vi "Versioned Write.vi"(9 "Path Stuff":T10 {"?"."Limits"."StoopidFast (fps)" min=0.0; "?"."Limits"."Jerk (fps^3)" min=0.0 step=1.0; "?"."Limits"."Accel (fps^2)" min=0.0; "?"."Limits"."Velocity (fps)" min=0.0; "?"."Overrides"."Angle Override" step=5.0; "?"."Overrides"."Velocity Override" step=5.0; "?"."Overrides"."Angular Override" step=5.0; "?"."Angular Limits"."Jerk (deg/s^3)" min=0.0 step=1.0; "?"."Angular Limits"."Accel (deg/s^2)" min=0.0; "?"."Angular Limits"."Velocity (deg/s)" min=0.0}, 10 "Filename":string, 11 "Bordeaux paths in":path) -> ()   [LabVIEW 2025]
uses:
  Types/Trajectory Data.ctl
  Types/Segment Type.ctl
  Types/Single Cmd Info.ctl
  <vilib>/picture/picture.llb/imagedata.ctl
  Types/Limits.ctl
  Types/Overrides.ctl
  Types/Angluar Limits.ctl
  Types/Drive Type.ctl
  Types/Path Type.ctl
panel:
  in  "?":T11
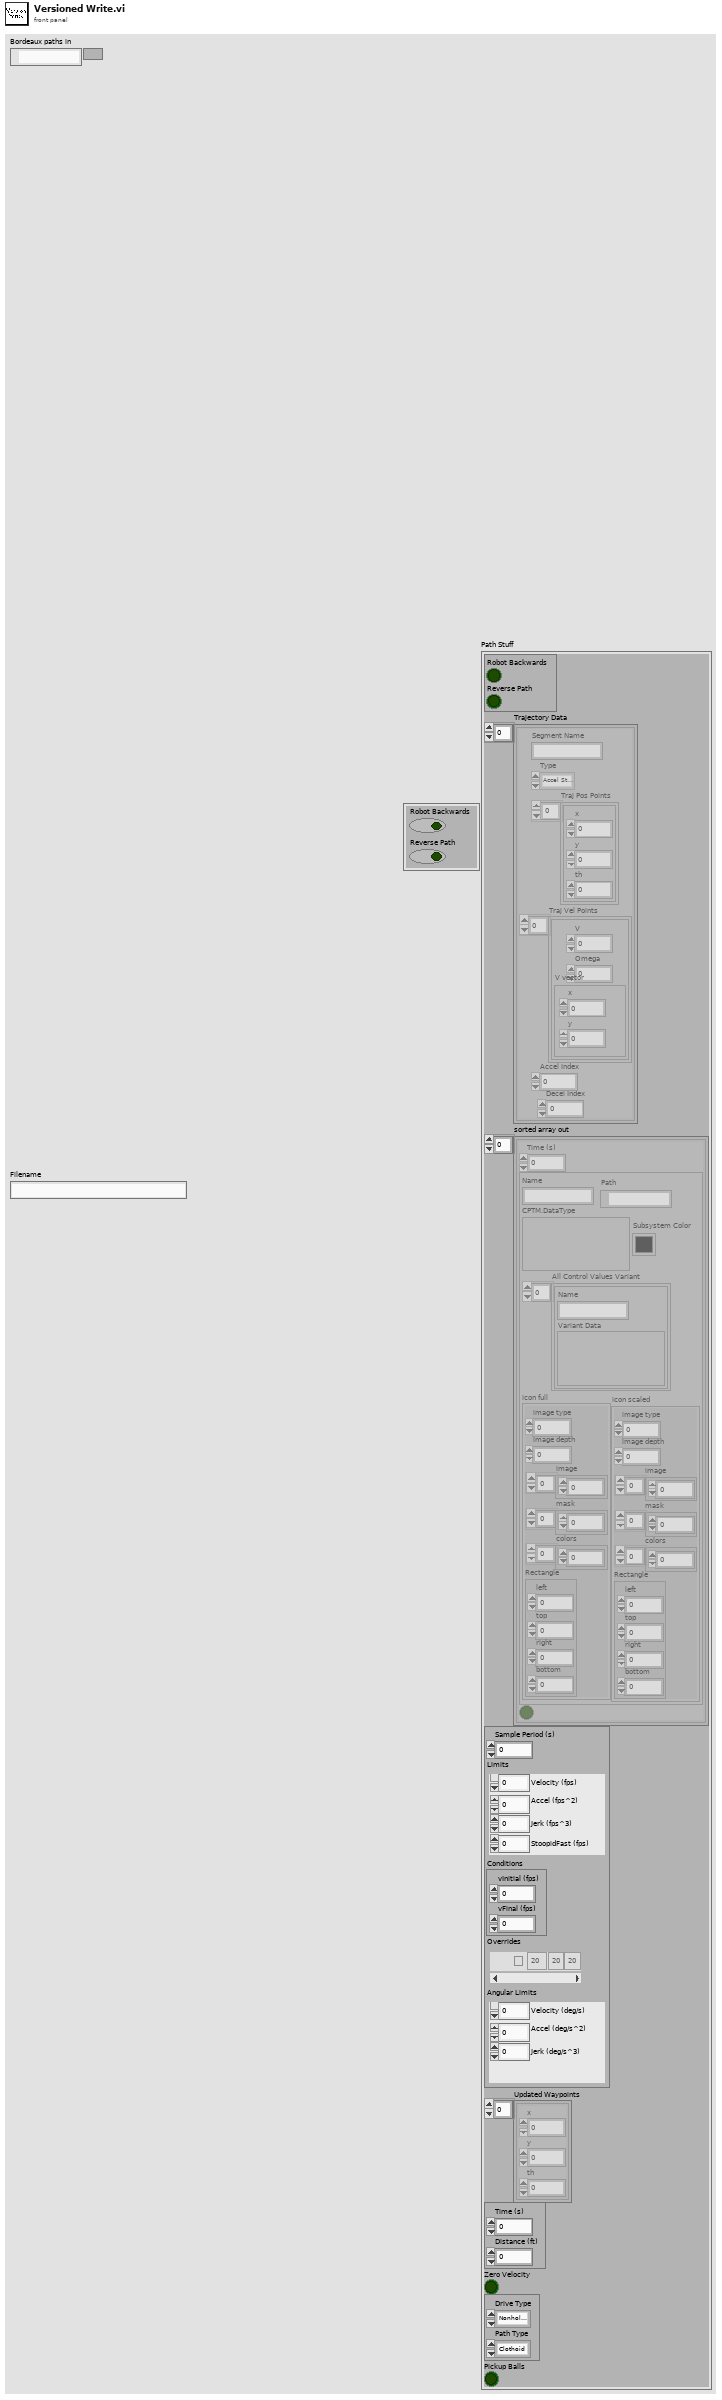
[diagram p1: front panel]
types:
  T1 = typedef "Trajectory Data.ctl" = cluster{"Segment Name":string, "Type":T2, "Traj Pos Points":cluster{"x":dbl, "y":dbl, "th":dbl}[], "Traj Vel Points":cluster{"V":dbl, "Omega":dbl, "V vector":cluster{"y":dbl, "x":dbl}}[], "Accel Index":i32, "Decel Index":i32}[]
  T2 = typedef "Segment Type.ctl" = enum16{"Accel Straight", "Const Straight", "Blend", "Circle", "Bezier"}
  T3 = typedef "Single Cmd Info.ctl" = cluster{"Name":string, "CPTM.DataType":variant, "All Control Values Variant":cluster{"Name":string, "Variant Data":variant}[], "icon full":T4, "icon scaled":T4, "Path":path, "Subsystem Color":u32}
  T4 = typedef "imagedata.ctl" = cluster{"image type":i32, "image depth":i32, "image":u8[], "mask":u8[], "colors":u32[], "Rectangle":cluster{"left":i16, "top":i16, "right":i16, "bottom":i16}}
  T5 = typedef "Limits.ctl" = cluster{"Velocity (fps)":dbl, "Accel (fps^2)":dbl, "Jerk (fps^3)":dbl, "StoopidFast (fps)":dbl}
  T6 = typedef "Overrides.ctl" = cluster{"Count":string, "Angular Override":dbl, "Enabled?":bool, "Velocity Override":dbl, "Angle Override":dbl}[]
  T7 = typedef "Angluar Limits.ctl" = cluster{"Velocity (deg/s)":dbl, "Accel (deg/s^2)":dbl, "Jerk (deg/s^3)":dbl}
  T8 = typedef "Drive Type.ctl" = enum16{"Nonholonomic", "Holonomic"}
  T9 = typedef "Path Type.ctl" = enum16{"Clothoid", "Bezier"}
  T10 = cluster{cluster{"Robot Backwards":bool, "Reverse Path":bool}, "Trajectory Data":T1, "sorted array out":cluster{"Time (s)":dbl, T3, bool}[], cluster{"Sample Period (s)":dbl, "Limits":T5, "Conditions":cluster{"vInitial (fps)":dbl, "vFinal (fps)":dbl}, "Overrides":T6, "Angular Limits":T7}, "Updated Waypoints":cluster{"x":dbl, "y":dbl, "th":dbl}[], cluster{"Time (s)":dbl, "Distance (ft)":dbl}, "Zero Velocity":bool, cluster{"Drive Type":T8, "Path Type":T9}, "Pickup Balls":bool}
  T11 = cluster{"Robot Backwards":bool, "Reverse Path":bool}
  T12 = cluster{"Sample Period (s)":dbl, "Limits":T5, "Conditions":cluster{"vInitial (fps)":dbl, "vFinal (fps)":dbl}, "Overrides":T6, "Angular Limits":T7}
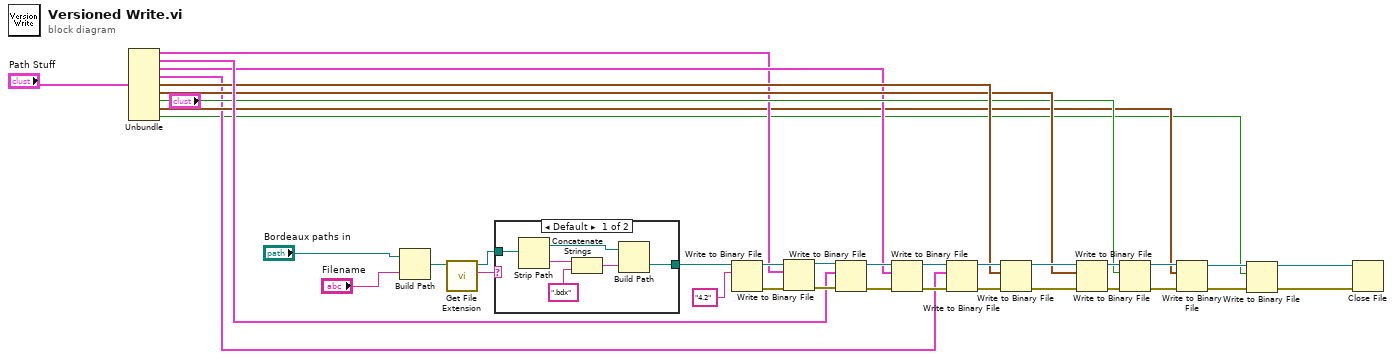
[diagram p0: block diagram]
diagram:
  n1 = Unbundle("Path Stuff") -> (w10:T11, "Trajectory Data"=w15:T1, "sorted array out"=w11:cluster{"Time (s)":dbl, T3, bool}[], w5:T12, "Updated Waypoints"=w14:cluster{"x":dbl, "y":dbl, "th":dbl}[], w13:cluster{"Time (s)":dbl, "Distance (ft)":dbl}, "Zero Velocity"=w12:bool, w6:cluster{"Drive Type":T8, "Path Type":T9}, "Pickup Balls"=w2:bool)
  n2 = Build Path(base path="Bordeaux paths in", name or relative path="Filename") -> (appended path=w33:path)
  n3 = call <vilib>:"Get File Extension.vi"("file"=w33) -> ("lowercase file extension"=w34:string, "dup file"=w35:path)  [unwired: 6 in, 3 out]
  n4 = case shown="Default" w34 {
    tunnel: w35 -> [w41 w43]
    tunnel: [w38 w43] -> w36
    frame Default {
      n5 = Strip Path(path=w41) -> (stripped path=w39:path, name=w40:string)
      n6 = Concatenate Strings(w40, ".bdx") -> (w37:string)
      n7 = Build Path(base path=w39, name or relative path=w37) -> (appended path=w38:path)
    }
    frame "bdx" {
    }
  }
  n8 = Write to Binary File(file (use dialog)=w36, data="4.2") -> (refnum out=w18:refnum<file>, error out=w24:errorcluster)  [unwired: 4 in, 1 out]
  n9 = Write to Binary File(file (use dialog)=w18, data=w10, error in=w24) -> (refnum out=w20:refnum<file>, error out=w25:errorcluster)  [unwired: 3 in, 1 out]
  n10 = Write to Binary File(file (use dialog)=w20, data=w15, error in=w25) -> (refnum out=w21:refnum<file>, error out=w26:errorcluster)  [unwired: 3 in, 1 out]
  n11 = Write to Binary File(file (use dialog)=w21, data=w11, error in=w26) -> (refnum out=w22:refnum<file>, error out=w27:errorcluster)  [unwired: 3 in, 1 out]
  n12 = Write to Binary File(file (use dialog)=w22, data=w5, error in=w27) -> (refnum out=w16:refnum<file>, error out=w28:errorcluster)  [unwired: 3 in, 1 out]
  n13 = Write to Binary File(file (use dialog)=w16, data=w14, error in=w28) -> (refnum out=w19:refnum<file>, error out=w29:errorcluster)  [unwired: 3 in, 1 out]
  n14 = Write to Binary File(file (use dialog)=w19, data=w13, error in=w29) -> (refnum out=w23:refnum<file>, error out=w30:errorcluster)  [unwired: 3 in, 1 out]
  n15 = Write to Binary File(file (use dialog)=w23, data=w12, error in=w30) -> (refnum out=w9:refnum<file>, error out=w8:errorcluster)  [unwired: 3 in, 1 out]
  n16 = Write to Binary File(file (use dialog)=w9, data=w6, error in=w8) -> (refnum out=w3:refnum<file>, error out=w7:errorcluster)  [unwired: 3 in, 1 out]
  n17 = Write to Binary File(file (use dialog)=w3, data=w2) -> (refnum out=w1:refnum<file>)  [unwired: 4 in, 2 out]
  n18 = Close File(refnum=w1, error in=w7) -> ()  [unwired: 2 out]
